vi "GT Helix XYRZWN.vi"(0 "cardNum":i16, 1 "crd":i16, 2 "x":i32, 3 "y":i32, 4 "z":i32, 5 "radius":dbl, 6 "circleDir":i16, 7 "error in (no error)":errorcluster caption="错误输入（无错误）", 8 "synVel":dbl, 9 "synAcc":dbl, 10 "velEnd":dbl, 11 "segNum":i32, 12 "fifo":i16) -> (20 "function return":i16, 27 "error out":errorcluster caption="错误输出")   [LabVIEW 2020, in "gts.lvlib"]
doc: "GT_API GT_HelixXYRZWN(short cardNum,short crd,long x,long y,long z,double radius,short circleDir,double synVel,double synAcc,double velEnd=0,long segNum=0,short fifo=0);"
uses:
  gts.lvlib
  dll/32bit/multi_card/gts.dll
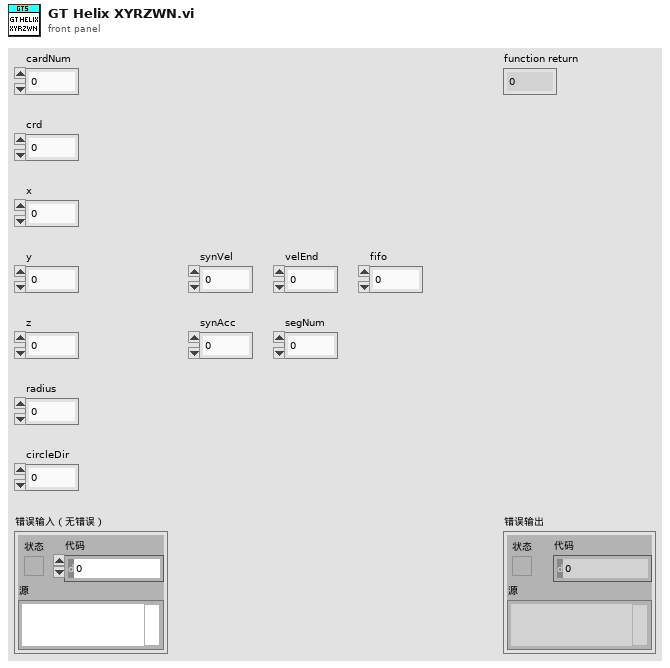
[diagram p1: front panel]
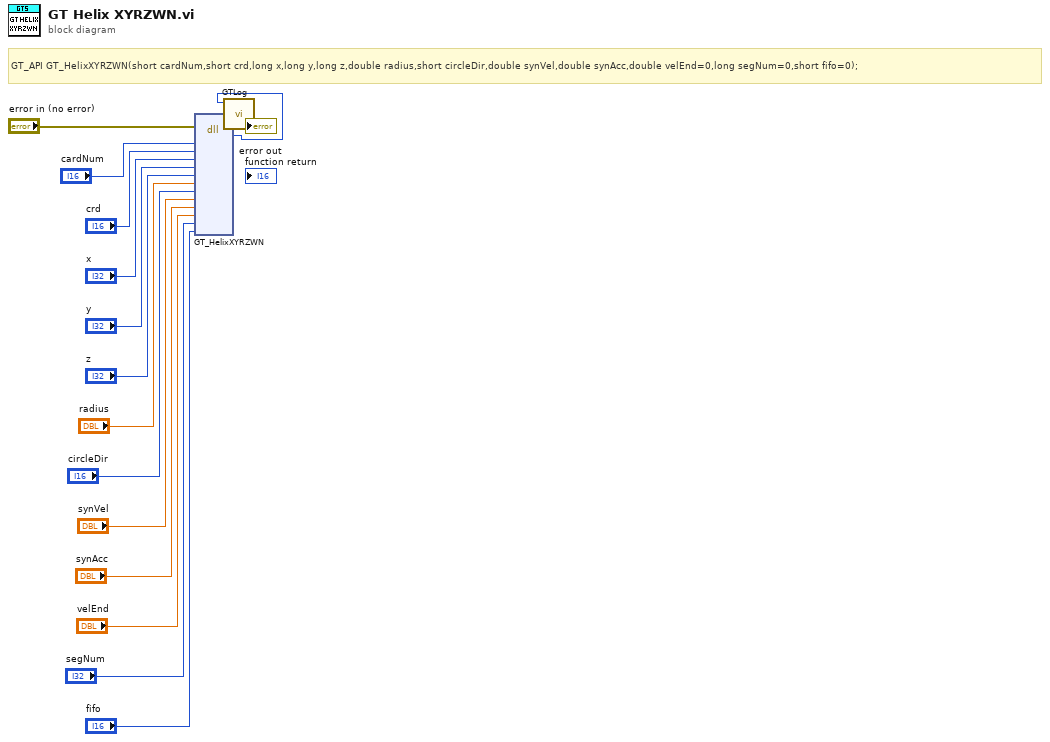
[diagram p0: block diagram]
diagram:
  # "GT_API GT_HelixXYRZWN(short cardNum,short crd,long x,long y,long z,double radius,short circleDir,double synVel,double synAcc,double velEnd=0,long segNum=0,short fifo=0);"
  n1 = dll-call lib="C:/1228/dll/32bit/multi_card/gts.dll" fn="GT_HelixXYRZWN"(error in="error in (no error)", "cardNum"="cardNum", "crd"="crd", "x"="x", "y"="y", "z"="z", "radius"="radius", "circleDir"="circleDir", "synVel"="synVel", "synAcc"="synAcc", "velEnd"="velEnd", "segNum"="segNum", "fifo"="fifo") -> (error out=w3:errorcluster, w1:i16)  [unwired: 14 in, 1 out]
  n2 = call "GTLog.vi"("error in (no error)"=w3, "Numeric"=w1) -> ("error out"=→"error out":errorcluster)  [unwired: 9 in]
